vi "AudioTest.Calculate Average Mag.vi"(10 "Average Level Calculation":T1={"Freq Start"=20.0, "Freq End"=20000.0}, 11 "Magnitude":cluster{"X":dbl[], "Y":dbl[]}) -> (3 "Average Mag":dbl)   [LabVIEW 2018]
uses:
  TypeDefs/AudioTest.Config, Average Level Config.ctl
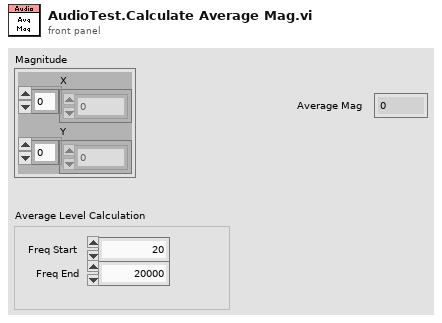
[diagram p1: front panel]
types:
  T1 = typedef "AudioTest.Config, Average Level Config.ctl" = cluster{"Freq Start":dbl, "Freq End":dbl}
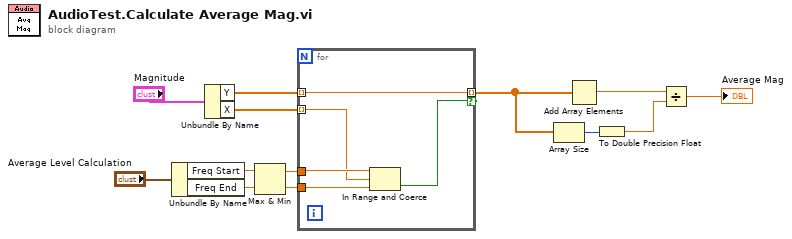
[diagram p0: block diagram]
diagram:
  n1 = Unbundle By Name("Average Level Calculation") -> ("Freq Start"=w9:dbl, "Freq End"=w8:dbl)
  n2 = Unbundle By Name("Magnitude") -> ("Y"=w11:dbl[], "X"=w12:dbl[])
  n3 = Max & Min(x=w9, y=w8) -> (max(x,y)=w7:dbl, min(x,y)=w6:dbl)
  n4 = for {
    tunnel: w12 -> [w16] mode=indexing
    tunnel: w11 -> [w15] mode=indexing
    tunnel: w7 -> [w18]
    tunnel: w6 -> [w17]
    tunnel: [w15] -> w5 mode=indexing if=w14
    n5 = In Range and Coerce(upper limit=w18, x=w16, lower limit=w17) -> (In Range?=w14:bool)  [unwired: 1 out]
  }
  n6 = Array Size(array=w5) -> (size(s)=w2:i32)
  n7 = Add Array Elements(numeric array=w5) -> (sum=w4:dbl)
  n8 = To Double Precision Float(number=w2) -> (double precision float=w3:dbl)
  n9 = Divide(x=w4, y=w3) -> (x/y=→"Average Mag":dbl)
